vi "Build G Object From Binary Stream.vi"(8 "error in (no error)":errorcluster, 9 ".NET Ads Binary Reader":refnum<k24>, 10 "Type Name":string, 11 "TwinCAT ADS in":refnum<class "TwinCAT ADS.lvclass">) -> (0 "error out":errorcluster, 2 "Value":variant, 3 "TwinCAT ADS out":refnum<class "TwinCAT ADS.lvclass">)   [LabVIEW 2018, in "TwinCAT ADS.lvclass"]
uses:
  TwinCAT ADS.lvclass
  TwinCAT.Ads
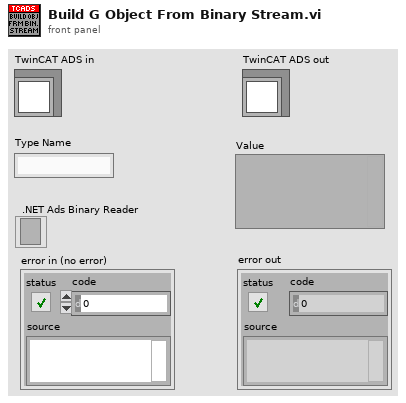
[diagram p1: front panel]
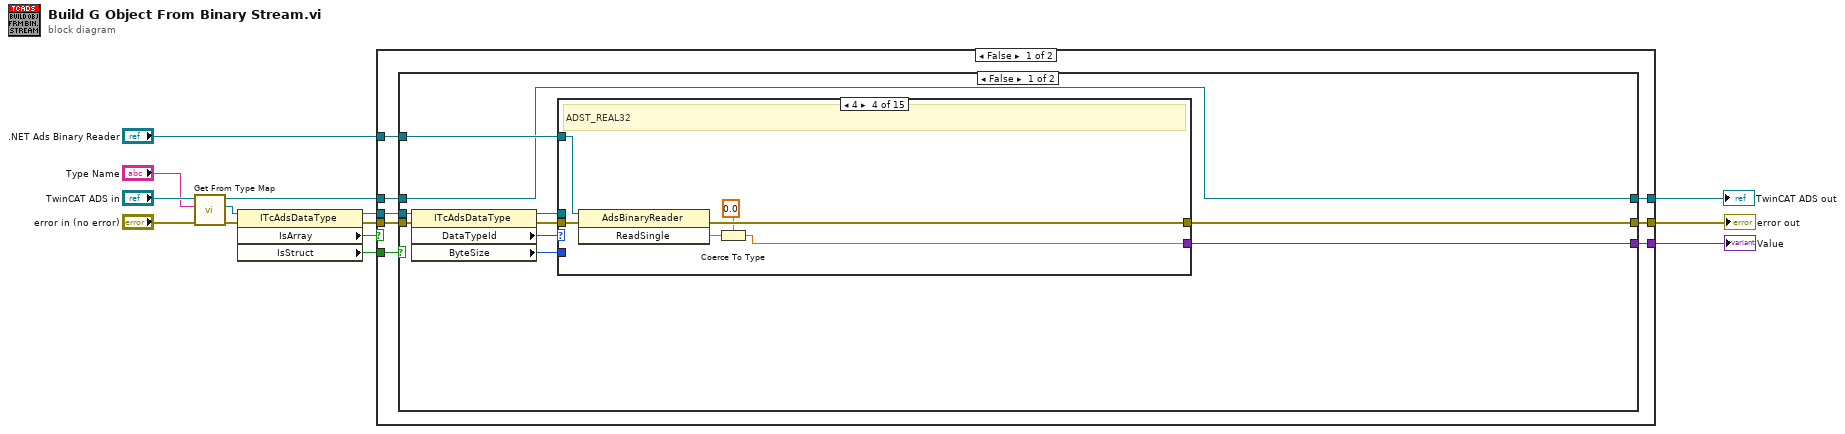
[diagram p0: block diagram]
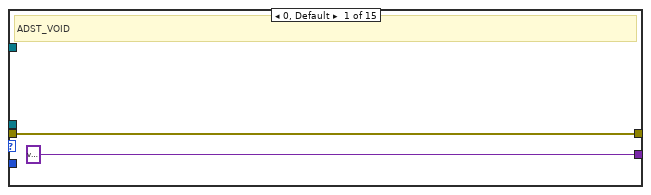
[diagram p2: hidden frame]
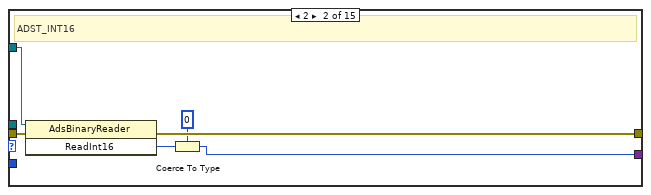
[diagram p3: hidden frame]
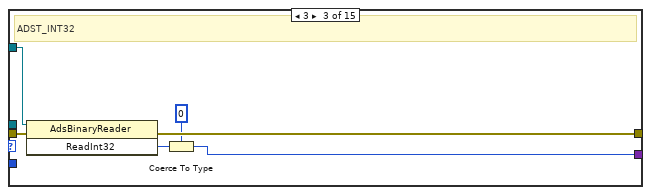
[diagram p4: hidden frame]
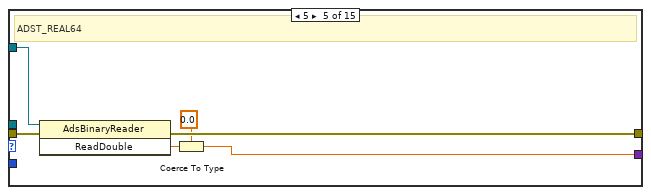
[diagram p5: hidden frame]
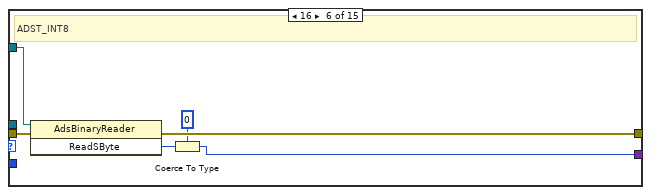
[diagram p6: hidden frame]
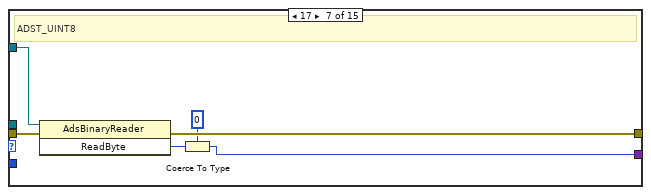
[diagram p7: hidden frame]
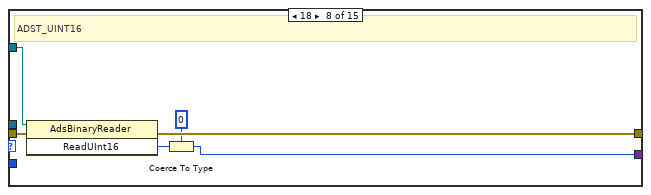
[diagram p8: hidden frame]
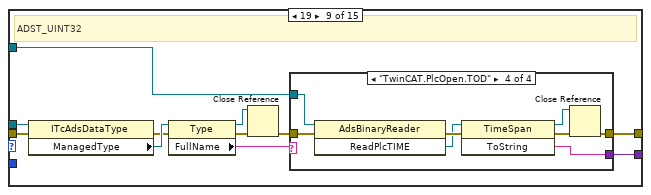
[diagram p9: hidden frame]
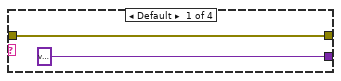
[diagram p10: hidden frame]
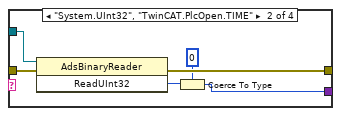
[diagram p11: hidden frame]
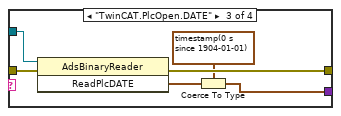
[diagram p12: hidden frame]
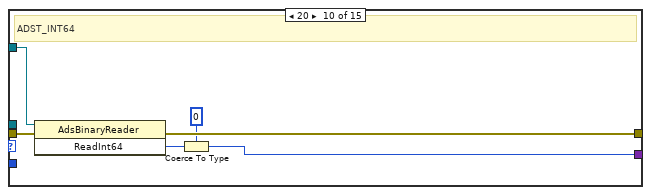
[diagram p13: hidden frame]
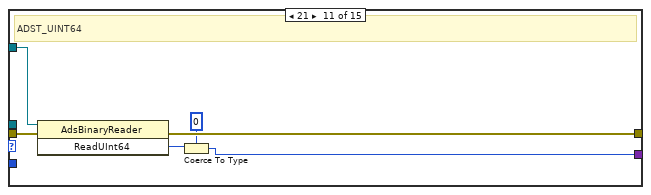
[diagram p14: hidden frame]
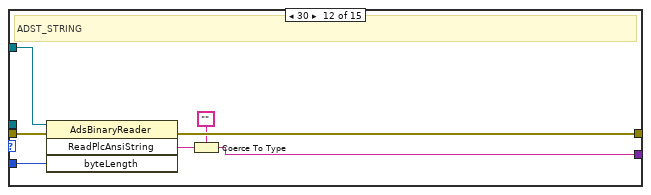
[diagram p15: hidden frame]
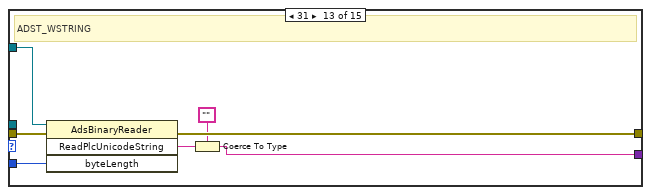
[diagram p16: hidden frame]
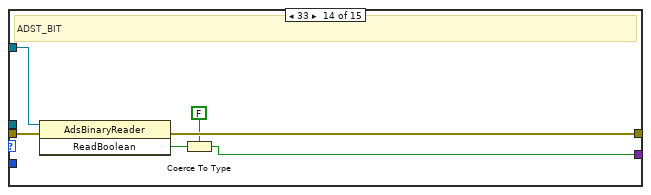
[diagram p17: hidden frame]
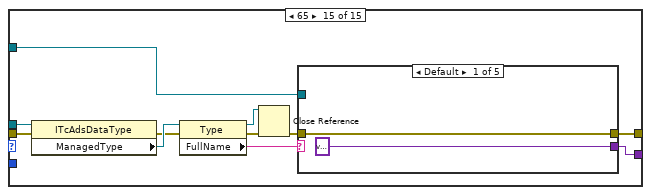
[diagram p18: hidden frame]
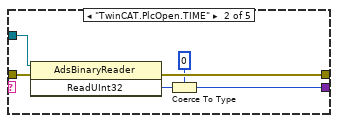
[diagram p19: hidden frame]
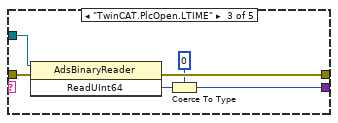
[diagram p20: hidden frame]
diagram:
  n1 = call "Get From Type Map.vi"("error in (no error)"="error in (no error)", "Type Name"="Type Name", "TwinCAT ADS in"="TwinCAT ADS in") -> ("error out"=w6:errorcluster, ".NET AdsDataType"=w5:refnum<k24>, "TwinCAT ADS out"=w7:refnum<class "TwinCAT ADS.lvclass">)  [unwired: 6 in]
  n2 = property class="ITcAdsDataType"(reference=w5, error in=w6) -> (reference out=w8:refnum<k24>, error out=w12:errorcluster, "IsArray"=w11:bool, "IsStruct"=w10:bool)
  n3 = case shown="False" w11 {
    tunnel: w12 -> [w22 w257]
    tunnel: w8 -> [w21 w256]
    tunnel: ".NET Ads Binary Reader" -> [w20 w260]
    tunnel: [w19 w259] -> w1
    tunnel: [w18 w258] -> w13
    tunnel: w10 -> [w17 _]
    tunnel: w7 -> [w16 w247]
    tunnel: [w15 w246] -> w9
    frame False {
      n4 = case shown="False" w17 {
        tunnel: w22 -> [w32 w198]
        tunnel: w21 -> [w31 w197]
        tunnel: w20 -> [w27 w192]
        tunnel: [w26 w187] -> w19
        tunnel: [w25 w186] -> w18
        tunnel: w16 -> [w23 w182]
        tunnel: [w23 w181] -> w15
        frame False {
          n5 = property class="ITcAdsDataType"(reference=w31, error in=w32) -> (reference out=w24:refnum<k24>, error out=w30:errorcluster, "DataTypeId"=w29:i32, "ByteSize"=w28:i32)
          n6 = case shown="4" w29 {
            tunnel: [variant w35 w41 w47 w53 w59 w65 w71 w84 w110 w116 w123 w130 w136 w145] -> w25
            tunnel: w30 -> [w33 w40 w46 w52 w58 w64 w70 w75 w79 w115 w121 w128 w135 w141 w144]
            tunnel: w28 -> [_ _ _ _ _ _ _ _ _ _ _ w126 w133 _ _]
            tunnel: w27 -> [_ w39 w45 w51 w57 w63 w69 w76 w83 w114 w120 w127 w134 w140 w147]
            tunnel: [w33 w38 w44 w50 w56 w62 w68 w74 w87 w113 w119 w125 w132 w139 w146] -> w26
            tunnel: w24 -> [_ _ _ _ _ _ _ _ w78 _ _ _ _ _ w143]
            frame 0, Default {
              # "ADST_VOID"
            }
            frame 2 {
              # "ADST_INT16"
              n7 = invoke class="AdsBinaryReader" method="ReadInt16"(reference=w39, error in=w40) -> (error out=w38:errorcluster, "ReadInt16"=w36:i16)  [unwired: 1 in, 1 out]
              n8 = Coerce To Type(0:w36, 1:i16 0) -> (2:w35:i16)
            }
            frame 3 {
              # "ADST_INT32"
              n9 = invoke class="AdsBinaryReader" method="ReadInt32"(reference=w45, error in=w46) -> (error out=w44:errorcluster, "ReadInt32"=w43:i32)  [unwired: 1 in, 1 out]
              n10 = Coerce To Type(0:w43, 1:0) -> (2:w41:i32)
            }
            frame 4 {
              # "ADST_REAL32"
              n11 = invoke class="AdsBinaryReader" method="ReadSingle"(reference=w51, error in=w52) -> (error out=w50:errorcluster, "ReadSingle"=w48:sgl)  [unwired: 1 in, 1 out]
              n12 = Coerce To Type(0:w48, 1:sgl 0.0) -> (2:w47:sgl)
            }
            frame 5 {
              # "ADST_REAL64"
              n13 = invoke class="AdsBinaryReader" method="ReadDouble"(reference=w57, error in=w58) -> (error out=w56:errorcluster, "ReadDouble"=w54:dbl)  [unwired: 1 in, 1 out]
              n14 = Coerce To Type(0:w54, 1:0.0) -> (2:w53:dbl)
            }
            frame 16 {
              # "ADST_INT8"
              n15 = invoke class="AdsBinaryReader" method="ReadSByte"(reference=w63, error in=w64) -> (error out=w62:errorcluster, "ReadSByte"=w60:i8)  [unwired: 1 in, 1 out]
              n16 = Coerce To Type(0:w60, 1:i8 0) -> (2:w59:i8)
            }
            frame 17 {
              # "ADST_UINT8"
              n17 = invoke class="AdsBinaryReader" method="ReadByte"(reference=w69, error in=w70) -> (error out=w68:errorcluster, "ReadByte"=w66:u8)  [unwired: 1 in, 1 out]
              n18 = Coerce To Type(0:w66, 1:u8 0) -> (2:w65:u8)
            }
            frame 18 {
              # "ADST_UINT16"
              n19 = invoke class="AdsBinaryReader" method="ReadUInt16"(reference=w76, error in=w75) -> (error out=w74:errorcluster, "ReadUInt16"=w72:u16)  [unwired: 1 in, 1 out]
              n20 = Coerce To Type(0:w72, 1:u16 0) -> (2:w71:u16)
            }
            frame 19 {
              # "ADST_UINT32"
              n21 = property class="ITcAdsDataType"(reference=w78, error in=w79) -> (error out=w77:errorcluster, "ManagedType"=w86:refnum<k24>)  [unwired: 1 out]
              n22 = property class="Type"(reference=w86, error in=w77) -> (reference out=w80:refnum<k24>, error out=w82:errorcluster, "FullName"=w85:string)
              n23 = Close Reference(reference=w80, error in (no error)=w82) -> (error out=w81:errorcluster)
              n24 = case shown="\"TwinCAT.PlcOpen.TOD\"" w85 {
                tunnel: [w89 w93 w99 w103] -> w87
                tunnel: w81 -> [w89 w95 w101 w109]
                tunnel: [variant ("ReadInt16") w90 w97 w105] -> w84
                tunnel: w83 -> [_ w94 w100 w108]
                frame Default {
                }
                frame "System.UInt32", "TwinCAT.PlcOpen.TIME" {
                  n25 = invoke class="AdsBinaryReader" method="ReadUInt32"(reference=w94, error in=w95) -> (error out=w93:errorcluster, "ReadUInt32"=w91:u32)  [unwired: 1 in, 1 out]
                  n26 = Coerce To Type(0:w91, 1:u32 0) -> (2:w90:u32)
                }
                frame "TwinCAT.PlcOpen.DATE" {
                  n27 = invoke class="AdsBinaryReader" method="ReadPlcDATE"(reference=w100, error in=w101) -> (error out=w99:errorcluster, "ReadPlcDATE"=w98:timestamp)  [unwired: 1 in, 1 out]
                  n28 = Coerce To Type(0:w98, 1:timestamp(0 s since 1904-01-01)) -> (2:w97:timestamp)
                }
                frame "TwinCAT.PlcOpen.TOD" {
                  n29 = invoke class="AdsBinaryReader" method="ReadPlcTIME"(reference=w108, error in=w109) -> (error out=w107:errorcluster, "ReadPlcTIME"=w106:refnum<k24>)  [unwired: 1 in, 1 out]
                  n30 = invoke class="TimeSpan" method="ToString"(reference=w106, error in=w107) -> (reference out=w102:refnum<k24>, error out=w104:errorcluster, "ToString"=w105:string)  [unwired: 1 in]
                  n31 = Close Reference(reference=w102, error in (no error)=w104) -> (error out=w103:errorcluster)
                }
              }
            }
            frame 20 {
              # "ADST_INT64"
              n32 = invoke class="AdsBinaryReader" method="ReadInt64"(reference=w114, error in=w115) -> (error out=w113:errorcluster, "ReadInt64"=w111:i64)  [unwired: 1 in, 1 out]
              n33 = Coerce To Type(0:w111, 1:i64 0) -> (2:w110:i64)
            }
            frame 21 {
              # "ADST_UINT64"
              n34 = invoke class="AdsBinaryReader" method="ReadUInt64"(reference=w120, error in=w121) -> (error out=w119:errorcluster, "ReadUInt64"=w117:u64)  [unwired: 1 in, 1 out]
              n35 = Coerce To Type(0:w117, 1:u64 0) -> (2:w116:u64)
            }
            frame 30 {
              # "ADST_STRING"
              n36 = invoke class="AdsBinaryReader" method="ReadPlcAnsiString"(reference=w127, error in=w128, "byteLength"=w126) -> (error out=w125:errorcluster, "ReadPlcAnsiString"=w124:string)  [unwired: 1 in, 2 out]
              n37 = Coerce To Type(0:w124, 1:"") -> (2:w123:string)
            }
            frame 31 {
              # "ADST_WSTRING"
              n38 = invoke class="AdsBinaryReader" method="ReadPlcUnicodeString"(reference=w134, error in=w135, "byteLength"=w133) -> (error out=w132:errorcluster, "ReadPlcUnicodeString"=w131:string)  [unwired: 1 in, 2 out]
              n39 = Coerce To Type(0:w131, 1:"") -> (2:w130:string)
            }
            frame 33 {
              # "ADST_BIT"
              n40 = invoke class="AdsBinaryReader" method="ReadBoolean"(reference=w140, error in=w141) -> (error out=w139:errorcluster, "ReadBoolean"=w138:bool)  [unwired: 1 in, 1 out]
              n41 = Coerce To Type(0:w138, 1:FALSE) -> (2:w136:bool)
            }
            frame 65 {
              n42 = property class="ITcAdsDataType"(reference=w143, error in=w144) -> (error out=w142:errorcluster, "ManagedType"=w152:refnum<k24>)  [unwired: 1 out]
              n43 = property class="Type"(reference=w152, error in=w142) -> (reference out=w150:refnum<k24>, error out=w151:errorcluster, "FullName"=w149:string)
              n44 = Close Reference(reference=w150, error in (no error)=w151) -> (error out=w148:errorcluster)
              n45 = case shown="Default" w149 {
                tunnel: w148 -> [w154 w160 w166 w170 w176]
                tunnel: w147 -> [_ w159 w165 w169 w173]
                tunnel: [w154 w158 w164 w168 w174] -> w146
                tunnel: [variant ("ReadInt16") w155 w161 w167 w175] -> w145
                frame Default {
                }
                frame "TwinCAT.PlcOpen.TIME" {
                  n46 = invoke class="AdsBinaryReader" method="ReadUInt32"(reference=w159, error in=w160) -> (error out=w158:errorcluster, "ReadUInt32"=w156:u32)  [unwired: 1 in, 1 out]
                  n47 = Coerce To Type(0:w156, 1:u32 0) -> (2:w155:u32)
                }
                frame "TwinCAT.PlcOpen.LTIME" {
                  n48 = invoke class="AdsBinaryReader" method="ReadUInt64"(reference=w165, error in=w166) -> (error out=w164:errorcluster, "ReadUInt64"=w162:u64)  [unwired: 1 in, 1 out]
                  n49 = Coerce To Type(0:w162, 1:u64 0) -> (2:w161:u64)
                }
                frame "TwinCAT.PlcOpen.DATE", "TwinCAT.PlcOpen.DT" {
                  n50 = invoke class="AdsBinaryReader" method="ReadPlcDATE"(reference=w169, error in=w170) -> (error out=w168:errorcluster, "ReadPlcDATE"=w172:timestamp)  [unwired: 1 in, 1 out]
                  n51 = Coerce To Type(0:w172, 1:timestamp(0 s since 1904-01-01)) -> (2:w167:timestamp)
                }
                frame "TwinCAT.PlcOpen.TOD" {
                  n52 = invoke class="AdsBinaryReader" method="ReadPlcTIME"(reference=w173, error in=w176) -> (error out=w180:errorcluster, "ReadPlcTIME"=w179:refnum<k24>)  [unwired: 1 in, 1 out]
                  n53 = invoke class="TimeSpan" method="ToString"(reference=w179, error in=w180) -> (reference out=w177:refnum<k24>, error out=w178:errorcluster, "ToString"=w175:string)  [unwired: 1 in]
                  n54 = Close Reference(reference=w177, error in (no error)=w178) -> (error out=w174:errorcluster)
                }
              }
            }
          }
        }
        frame True {
          n55 = property class="AdsBinaryReader"(reference=w192) -> (reference out=w190:refnum<k24>, "BaseStream"=w191:refnum<k24>)  [unwired: 1 in, 1 out]
          n56 = property class="ITcAdsDataType"(reference=w197, error in=w198) -> (error out=w196:errorcluster, "SubItems"=w183:refnum<k24>)  [unwired: 1 out]
          n57 = property class="ReadOnlySubItemCollection"(reference=w183, error in=w196) -> (reference out=w194:refnum<k24>, error out=w195:errorcluster, "Count"=w193:i32)
          n58 = for {
            N: w193 -> [_]
            tunnel: w194 -> [w218]
            tunnel: w190 -> [w203]
            shift-right: [w205] -> w184
            shift-left: w195 -> [w219]
            shift-right: [w215] -> w189
            shift-left: w191 -> [w216]
            tunnel: [w204] -> w188 mode=indexing
            tunnel: [w202] -> w185 mode=indexing
            shift-right: [w213] -> _
            shift-left: _ -> [w212]
            shift-right: [w214] -> _
            shift-left: _ -> [w211]
            shift-right: [w201] -> w181
            shift-left: w182 -> [w220]
            i -> [w217]
            n59 = invoke class="ReadOnlySubItemCollection" method="get_Item"(reference=w218, error in=w219, "index"=w217) -> (error out=w210:errorcluster, "get_Item"=w209:refnum<k24>)  [unwired: 1 in, 2 out]
            n60 = property class="ITcAdsSubItem"(reference=w209, error in=w210) -> (reference out=w202:refnum<k24>, error out=w208:errorcluster, "Offset"=w207:i32, "ByteSize"=w206:i32, "Name"=w200:string)
            n61 = case shown="1.." w217 {
              tunnel: w208 -> [w224 w225 w242]
              tunnel: w216 -> [w223 w228 w241]
              tunnel: [w224 w225 w240] -> w199
              tunnel: [w223 w228 w238] -> w215
              tunnel: [w221 w226 w237] -> w214
              tunnel: [w222 w227 w233] -> w213
              tunnel: w212 -> [w222 _ w232]
              tunnel: w211 -> [w221 _ w231]
              tunnel: w207 -> [_ w227 w233]
              tunnel: w206 -> [_ w226 w237]
              frame Default {
              }
              frame 0 {
              }
              frame 1.. {
                n62 = property class="Stream"(reference=w241, error in=w242) -> (reference out=w239:refnum<k24>, error out=w235:errorcluster, "Position"=w236:i64)
                n63 = Add(x=w232, y=w231) -> (x+y=w230:i32)
                n64 = Subtract(x=w233, y=w230) -> (x-y=w229:i32)
                n65 = Add(x=w236, y=w229) -> (x+y=w234:i64)
                n66 = property class="Stream"(reference=w239, error in=w235, "Position"=w234) -> (reference out=w238:refnum<k24>, error out=w240:errorcluster)
              }
            }
            n67 = call "Build G Object From Binary Stream.vi"("error in (no error)"=w199, ".NET Ads Binary Reader"=w203, "Type Name"=w200, "TwinCAT ADS in"=w220) -> ("error out"=w205:errorcluster, "Value"=w204:variant, "TwinCAT ADS out"=w201:refnum<class "TwinCAT ADS.lvclass">)  [unwired: 5 in]
          }
          n68 = Close Reference(reference=w185) -> ()  [unwired: 1 in, 1 out]
          n69 = Close Reference(reference=w189) -> ()  [unwired: 1 in, 1 out]
          n70 = call "Array of Variants to Cluster Variant.vi"("error in (no error)"=w184, "[Variant]"=w188) -> ("error out"=w187:errorcluster, "Cluster Variant"=w186:variant)  [unwired: 8 in]
          n71 = Close Reference(reference=w183, error in (no error)=w184) -> ()  [unwired: 1 out]
        }
      }
    }
    frame True {
      n72 = property class="ITcAdsDataType"(reference=w256, error in=w257) -> (error out=w255:errorcluster, "Dimensions"=w254:refnum<k24>, "BaseType"=w245:refnum<k24>)  [unwired: 1 out]
      n73 = property class="ReadOnlyDimensionCollection"(reference=w254, error in=w255) -> (reference out=w250:refnum<k24>, error out=w249:errorcluster, "ElementCount"=w253:i32)
      n74 = property class="ITcAdsDataType"(reference=w245) -> (reference out=w244:refnum<k24>, "Name"=w243:string)  [unwired: 1 in, 1 out]
      n75 = Close Reference(reference=w244) -> ()  [unwired: 1 in, 1 out]
      n76 = Close Reference(reference=w250, error in (no error)=w249) -> (error out=w248:errorcluster)
      n77 = for {
        N: w253 -> [_]
        shift-right: [w266] -> w252
        shift-left: w248 -> [w264]
        tunnel: w260 -> [w267]
        tunnel: [w265] -> w251 mode=indexing
        shift-right: [w262] -> w246
        shift-left: w247 -> [w263]
        tunnel: w243 -> [w261]
        n78 = call "Build G Object From Binary Stream.vi"("error in (no error)"=w264, ".NET Ads Binary Reader"=w267, "Type Name"=w261, "TwinCAT ADS in"=w263) -> ("error out"=w266:errorcluster, "Value"=w265:variant, "TwinCAT ADS out"=w262:refnum<class "TwinCAT ADS.lvclass">)  [unwired: 5 in]
      }
      n79 = call "Array of Variants to Array Variant.vi"("error in (no error)"=w252, "[Variant]"=w251) -> ("error out"=w259:errorcluster, "Array Variant"=w258:variant)  [unwired: 8 in]
    }
  }
  "Value" <- w13
  "error out" <- w1
  "TwinCAT ADS out" <- w9
